vi "Update from Bool.vi"(5 "True String (True)":string="True", 6 "Timestamp (Now)":dbl, 7 "False String (False)":string="False", 8 "error in (no error)":errorcluster, 10 "Bool":bool, 11 "StringChannel in":refnum<class "Channel STR.lvclass">) -> (0 "error out":errorcluster, 3 "StringChannel out":refnum<class "Channel STR.lvclass">)   [LabVIEW 2020, in "Vecto.lvlib" / "Channel STR.lvclass"]
uses:
  Channel STR.lvclass
  Channel STR.lvclass/Channel STR.ctl
  Group STR/Group STR.lvclass
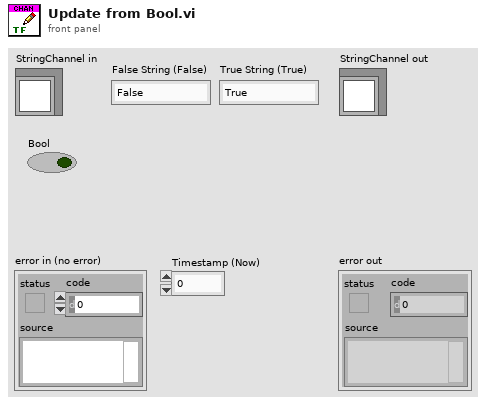
[diagram p1: front panel]
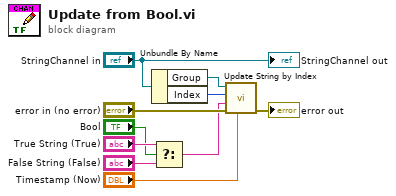
[diagram p0: block diagram]
diagram:
  n1 = Unbundle By Name("StringChannel in") -> ("Group"=w6:refnum<class "Group STR.lvclass">, "Index"=w7:i32)
  n2 = Select(t="True String (True)", s="Bool", f="False String (False)") -> (s? t:f=w1:string)
  n3 = call "Update String by Index.vi"("Timestamp (Now)"="Timestamp (Now)", "error in (no error)"="error in (no error)", "String"=w1, "Index"=w7, "StringGroup in"=w6) -> ("error out"=→"error out":errorcluster)  [unwired: 5 in, 1 out]
  "StringChannel out" <- "StringChannel in"
